vi "Write.vi"(6 "Append Index":i32, 8 "error in (no error)":errorcluster, 9 "Notes":string, 10 "Data (Dictionary)":T1[](array[typedef]), 11 "Data.HDF5 in":refnum<class "Data.HDF5.lvclass">) -> (0 "error out":errorcluster, 3 "Data.HDF5 out":refnum<class "Data.HDF5.lvclass">, 5 "Path out":path)   [LabVIEW 2019, in "Data.HDF5.lvclass"]
uses:
  Data.HDF5.lvclass
  Data/Data.lvclass
  C:/user/patrick/git/LV-to-ITX/src/Data/Data.lvclass
  Data/Typedefs/Dictionary--cluster.ctl
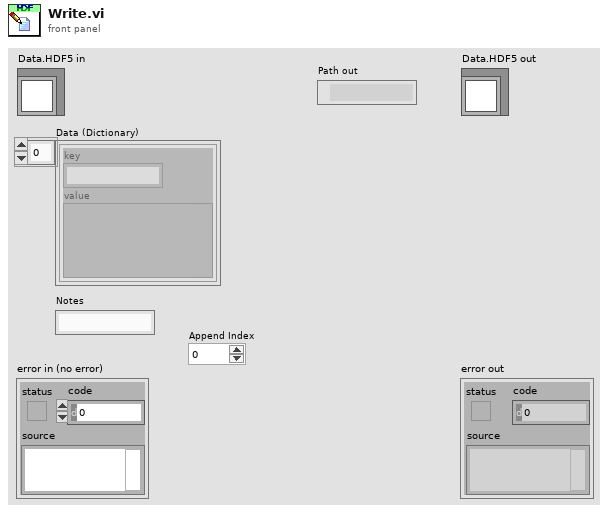
[diagram p1: front panel]
types:
  T1 = typedef "Data.lvclass/Dictionary--cluster.ctl" = cluster{"key":string, "value":variant}
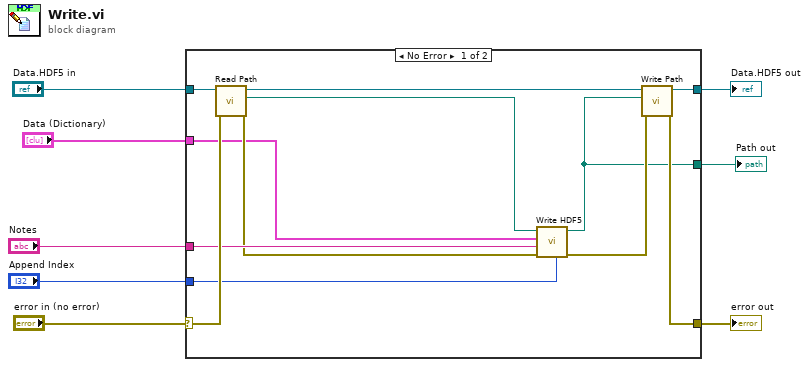
[diagram p0: block diagram]
diagram:
  n1 = case shown="No Error" "error in (no error)" {
    selector: "error in (no error)" -> [w19 w22]
    tunnel: [w17 w22] -> w6
    tunnel: "Data.HDF5 in" -> [w20 w21]
    tunnel: [w18 w21] -> w5
    tunnel: "Notes" -> [w14 _]
    tunnel: "Data (Dictionary)" -> [w12 _]
    tunnel: [w10 _] -> w2
    tunnel: "Append Index" -> [w9 _]
    frame No Error {
      n2 = call "Read Path.vi"("error in (no error)"=w19, "Data Save"=w20) -> ("error out"=w13:errorcluster, "Path"=w11:path, "Data Save out"=w16:refnum<class "Data.HDF5.lvclass">)  [unwired: 7 in]
      n3 = call "Write HDF5.vi"("Append (0=F)"=w9, "error in (no error)"=w13, "Notes"=w14, "Data (Dictionary)"=w12, "path"=w11) -> ("error out"=w15:errorcluster, "path out"=w10:path)  [unwired: 5 in]
      n4 = call "Write Path.vi"("error in (no error)"=w15, "Path"=w10, "Data Save"=w16) -> ("error out"=w17:errorcluster, "Data Save out"=w18:refnum<class "Data.HDF5.lvclass">)  [unwired: 7 in]
    }
    frame Error {
    }
  }
  "error out" <- w6
  "Data.HDF5 out" <- w5
  "Path out" <- w2
